vi "niDTS WLAN Dut Initialize.vi"(0 "Session Name ()":string, 2 "WLAN Dut Object Type":refnum<class "niDTS WLAN Dut.lvclass">, 5 "Comm Handle":T2, 7 "Logger":T1, 11 "error in (no error)":errorcluster) -> (4 "WLAN Dut Handle out":T3, 15 "error out":errorcluster)   [LabVIEW 2015, in "niDTS WLAN.lvlib"]
uses:
  niDTS WLAN.lvlib
  Includes/niDTS WLAN Dut INC Handle.ctl
  Objects/BASE_class/niDTS WLAN Dut.lvclass
  Framework/Comm/Includes/niDTS Comm INC Handle.ctl
  Framework/Comm/Objects/BASE_class/niDTS Comm.lvclass
  Framework/Logger/Includes/niDTS Logger INC Handle.ctl
  Framework/Logger/Objects/BASE_class/niDTS Logger.lvclass
  Framework/Session/Objects/BASE_class/niDTS Session.lvclass
  Framework/niDTS Framework.lvlib
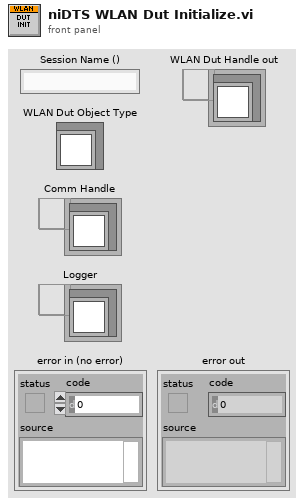
[diagram p1: front panel]
types:
  T1 = typedef "niDTS Framework.lvlib/niDTS Logger INC Handle.ctl" = refnum<data-value>
  T2 = typedef "niDTS Framework.lvlib/niDTS Comm INC Handle.ctl" = refnum<data-value>
  T3 = typedef "niDTS WLAN.lvlib/niDTS WLAN Dut INC Handle.ctl" = refnum<data-value>
  T4 = typedef "niDTS Framework.lvlib/niDTS Session INC Handle.ctl" = refnum<data-value>
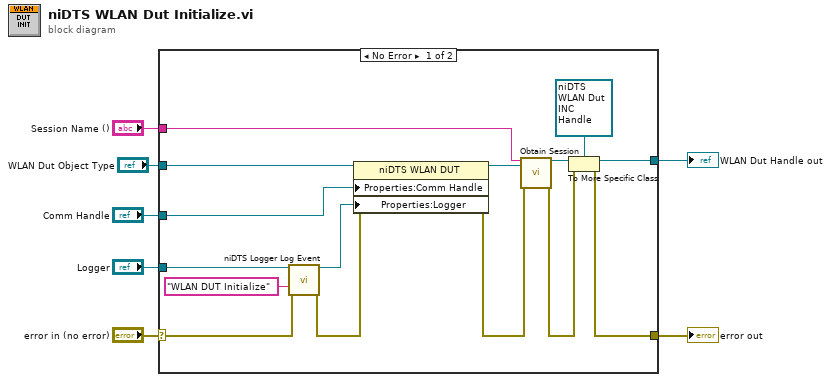
[diagram p0: block diagram]
diagram:
  n1 = case shown="No Error" "error in (no error)" {
    selector: "error in (no error)" -> [w11 w23]
    tunnel: "Session Name ()" -> [w9 _]
    tunnel: [w16 w23] -> w6
    tunnel: [w13 _] -> w4
    tunnel: "Comm Handle" -> [w22 _]
    tunnel: "Logger" -> [w21 _]
    tunnel: "WLAN Dut Object Type" -> [w8 _]
    frame No Error {
      n2 = call "niDTS Logger Log Event.vi"("Logger Handle"=w21, "Source/Location"="WLAN DUT Initialize", "error in (no error)"=w11) -> ("Logger Handle out"=w10:T1, "error out"=w17:errorcluster)  [unwired: 10 in, 1 out]
      n3 = property class="niDTS WLAN DUT"(reference=w8, error in=w17, "Properties:Comm Handle"=w22, "Properties:Logger"=w10) -> (reference out=w19:refnum<class "niDTS WLAN Dut.lvclass">, error out=w14:errorcluster)
      n4 = call "Obtain Session.vi"("Session Name ()"=w9, "OBJ - Session"=w19, "error in (no error)"=w14) -> ("Session Handle"=w20:T4, "error out"=w15:errorcluster)  [unwired: 10 in, 1 out]
      n5 = To More Specific Class(target class=T3 refnum ("WLAN Dut Handle"), reference=w20, error in=w15) -> (specific class reference=w13:T3, error out=w16:errorcluster)
    }
    frame Error {
    }
  }
  "error out" <- w6
  "WLAN Dut Handle out" <- w4
